vi "Globals.vi"() -> ()   [LabVIEW 2009]
panel:
  out "newSetpointCommand":bool
  out "busy":bool
  in  "channelInt":i32
  in  "rampRate":dbl
  in  "rampAmplitude":dbl
  in  "setpointTime":dbl
  in  "setpoint":dbl
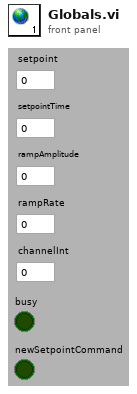
[diagram p1: front panel]
diagram:
